vi "Close Connection.vi"(8 "error in (no error)":errorcluster, 11 "object in":refnum<class "Simulado.lvclass">) -> (0 "error out":errorcluster, 3 "object out":refnum<class "Simulado.lvclass">)   [LabVIEW 2020, in "Simulado.lvclass"]
uses:
  Simulado.lvclass
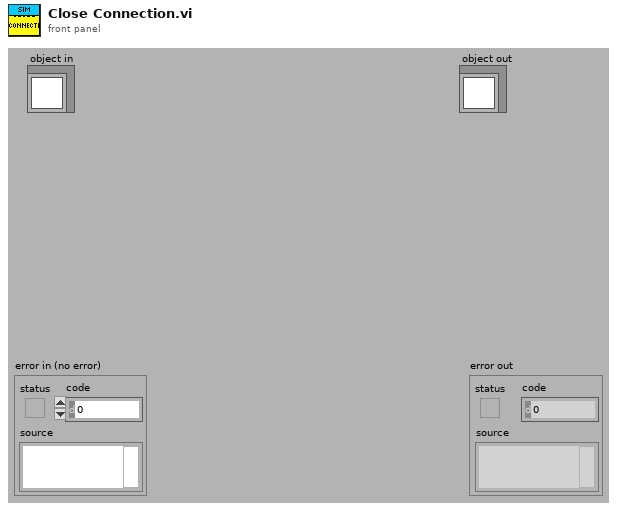
[diagram p1: front panel]
types:
  T1 = enum16{"Get Parameters", "Set Parameters", "Reset"}
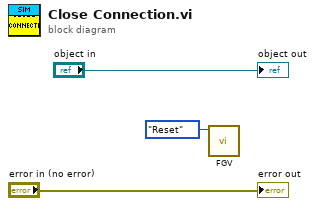
[diagram p0: block diagram]
diagram:
  n1 = call "FGV.vi"("Función"=T1."Reset") -> ()  [unwired: 10 in, 1 out]
  "error out" <- "error in (no error)"
  "object out" <- "object in"
